vi "GetProperties.vi"(8 "error in":errorcluster, 11 "Control in":refnum<class "Control.lvclass">) -> (0 "error out":errorcluster, 3 "Control out":refnum<class "Control.lvclass">)   [LabVIEW 2014, in "Control.lvclass"]
uses:
  Control.lvclass
  Control.lvclass/Control.ctl
  GObject/GObject.lvclass
  Text/Text.lvclass
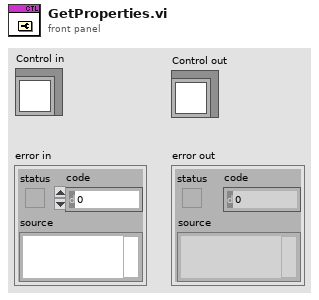
[diagram p1: front panel]
types:
  T1 = enum8{"Enabled", "Disabled", "Disabled and Grayed Out"}
  T2 = cluster{"Can Grow Horiz":bool, "Can Grow Vert":bool, "Min Horiz":i16, "Min Vert":i16, "Max Horiz":i16, "Max Vert":i16}
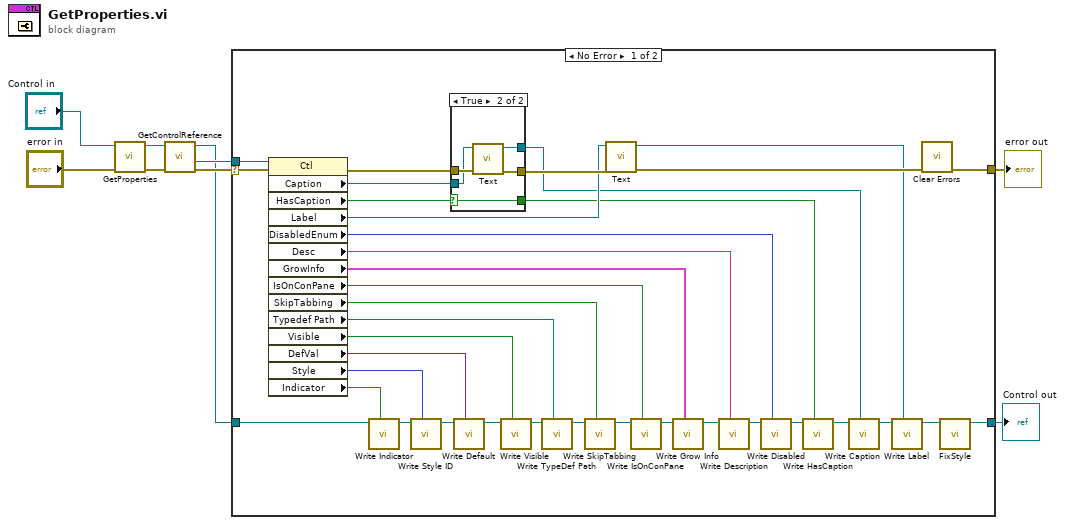
[diagram p0: block diagram]
diagram:
  n1 = call-parent "GetProperties.vi"("error in"="error in", "GObject in"="Control in") -> ("error out"=w3:errorcluster, "GObject out"=w4:refnum<class "Control.lvclass">)  [unwired: 8 in]
  n2 = call "GetControlReference.vi"("error in"=w3, "Control in"=w4) -> ("error out"=w8:errorcluster, "control reference"=w7:refnum<vi>, "Control out"=w6:refnum<class "Control.lvclass">)  [unwired: 7 in]
  n3 = case shown="No Error" w8 {
    selector: w8 -> [w46 w55]
    tunnel: [w12 w55] -> w9
    tunnel: w7 -> [w45 _]
    tunnel: w6 -> [w13 w54]
    tunnel: [w10 w54] -> w5
    frame No Error {
      n4 = property class="Ctl"(reference=w45, error in=w46) -> (error out=w44:errorcluster, "Caption"=w43:refnum<vi>, "HasCaption"=w40:bool, "Label"=w39:refnum<vi>, "DisabledEnum"=w24:T1, "Desc"=w28:string, "GrowInfo"=w30:T2, "IsOnConPane"=w32:bool, "SkipTabbing"=w34:bool, "Typedef Path"=w36:path, "Visible"=w38:bool, "DefVal"=w26:variant, "Style"=w16:u32, "Indicator"=w14:bool)  [unwired: 1 out]
      n5 = call "Write Indicator.vi"("Indicator"=w14, "Control in"=w13) -> ("Control out"=w15:refnum<class "Control.lvclass">)  [unwired: 7 in]
      n6 = call "Write Style ID.vi"("Style ID"=w16, "Control in"=w15) -> ("Control out"=w17:refnum<class "Control.lvclass">)  [unwired: 7 in]
      n7 = case shown="True" w40 {
        selector: w40 -> [w47 w49]
        tunnel: w44 -> [w48 w53]
        tunnel: w43 -> [_ w52]
        tunnel: [w48 w51] -> w41
        tunnel: [_ w50] -> w20
        tunnel: [w47 w49] -> w22
        frame False {
        }
        frame True {
          n8 = call "Text.vi"("error in"=w53, "Gen Refnum"=w52) -> ("error out"=w51:errorcluster, "Text out"=w50:refnum<class "Text.lvclass">)  [unwired: 8 in]
        }
      }
      n9 = call "Write Default.vi"("Default"=w26, "Control in"=w17) -> ("Control out"=w27:refnum<class "Control.lvclass">)  [unwired: 7 in]
      n10 = call "Write Visible.vi"("Visible"=w38, "Control in"=w27) -> ("Control out"=w37:refnum<class "Control.lvclass">)  [unwired: 7 in]
      n11 = call "Write TypeDef Path.vi"("TypeDef Path"=w36, "Control in"=w37) -> ("Control out"=w35:refnum<class "Control.lvclass">)  [unwired: 7 in]
      n12 = call "Write SkipTabbing.vi"("SkipTabbing"=w34, "Control in"=w35) -> ("Control out"=w33:refnum<class "Control.lvclass">)  [unwired: 7 in]
      n13 = call "Text.vi"("error in"=w41, "Gen Refnum"=w39) -> ("error out"=w42:errorcluster, "Text out"=w18:refnum<class "Text.lvclass">)  [unwired: 8 in]
      n14 = call "Write IsOnConPane.vi"("IsOnConPane"=w32, "Control in"=w33) -> ("Control out"=w31:refnum<class "Control.lvclass">)  [unwired: 7 in]
      n15 = call "Write Grow Info.vi"("Grow Info"=w30, "Control in"=w31) -> ("Control out"=w29:refnum<class "Control.lvclass">)  [unwired: 7 in]
      n16 = call "Write Description.vi"("Description"=w28, "Control in"=w29) -> ("Control out"=w25:refnum<class "Control.lvclass">)  [unwired: 7 in]
      n17 = call "Write Disabled.vi"("Disabled"=w24, "Control in"=w25) -> ("Control out"=w23:refnum<class "Control.lvclass">)  [unwired: 7 in]
      n18 = call "Write HasCaption.vi"("HasCaption"=w22, "Control in"=w23) -> ("Control out"=w21:refnum<class "Control.lvclass">)  [unwired: 7 in]
      n19 = call "Write Caption.vi"("Caption"=w20, "Control in"=w21) -> ("Control out"=w19:refnum<class "Control.lvclass">)  [unwired: 7 in]
      n20 = call "Write Label.vi"("Label"=w18, "Control in"=w19) -> ("Control out"=w11:refnum<class "Control.lvclass">)  [unwired: 7 in]
      n21 = call <vilib>:"Clear Errors.vi"("error in (no error)"=w42) -> ("error out"=w12:errorcluster)  [unwired: 5 in, 1 out]
      n22 = call "FixStyle.vi"("Control in"=w11) -> ("Control out"=w10:refnum<class "Control.lvclass">)  [unwired: 10 in]
    }
    frame Error {
    }
  }
  "error out" <- w9
  "Control out" <- w5
